vi "Find_array_index.vi"(5 "TIME MARGIN":dbl format="%.2f", 7 "AT 2 index":i32, 8 "AT 2 array":dbl[](array[numeric]) format="%.3f", 9 "AT 1 index":i32, 10 "AT 1 array":dbl[](array[numeric]) format="%.3f") -> (0 "AT 2 index out":i32, 3 "Found matching Element in array 2":bool)   [LabVIEW 2010]
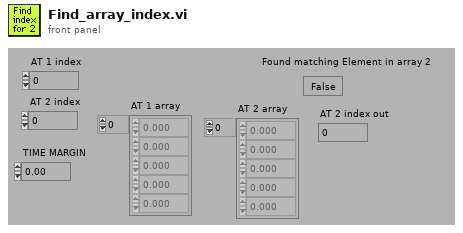
[diagram p1: front panel]
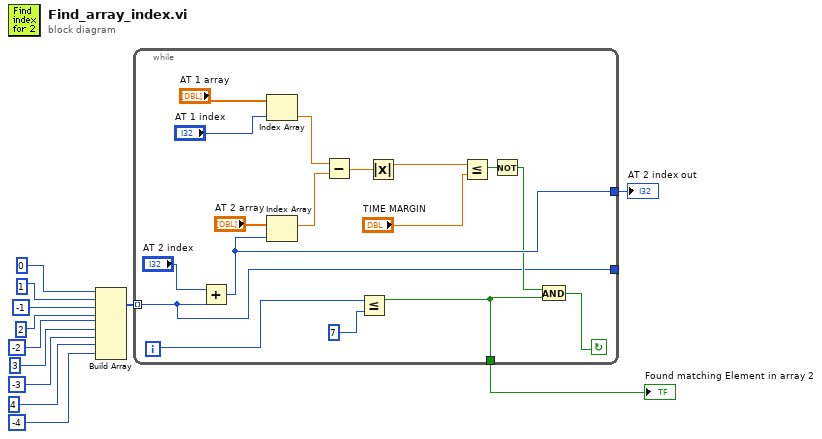
[diagram p0: block diagram]
diagram:
  n1 = Build Array(0, 1, -1, 2, -2, 3, -3, 4, -4) -> (w7:i32[])
  n2 = while {
    tunnel: [w15] -> _
    tunnel: w7 -> [w15] mode=indexing
    tunnel: [w17] -> w2
    tunnel: [w22] -> w1
    i -> [w16]
    stop <- w18 continue-if-true
    n3 = Add(x="AT 2 index", y=w15) -> (x+y=w22:i32)
    n4 = Index Array(array="AT 1 array", index="AT 1 index") -> (element=w28:dbl)
    n5 = Index Array(array="AT 2 array", index=w22) -> (element=w29:dbl)
    n6 = Subtract(x=w28, y=w29) -> (x-y=w27:dbl)
    n7 = Less Or Equal?(x=w16, y=7) -> (x <= y?=w17:bool)
    n8 = Absolute Value(x=w27) -> (abs(x)=w23:dbl)
    n9 = Less Or Equal?(x=w23, y="TIME MARGIN") -> (x <= y?=w20:bool)
    n10 = Not(x=w20) -> (.not. x?=w19:bool)
    n11 = And(x=w19, y=w17) -> (x .and. y?=w18:bool)
  }
  "AT 2 index out" <- w1
  "Found matching Element in array 2" <- w2
